vi "parse load from file.vi"(8 "error in":errorcluster, 11 "message data":string) -> (0 "error out":errorcluster, 2 "targets to load":string[](array[string]), 3 "path":path)   [LabVIEW 2013, in "module execution process.lvlib"]
uses:
  module execution process.lvlib
  tokenized path.ctl
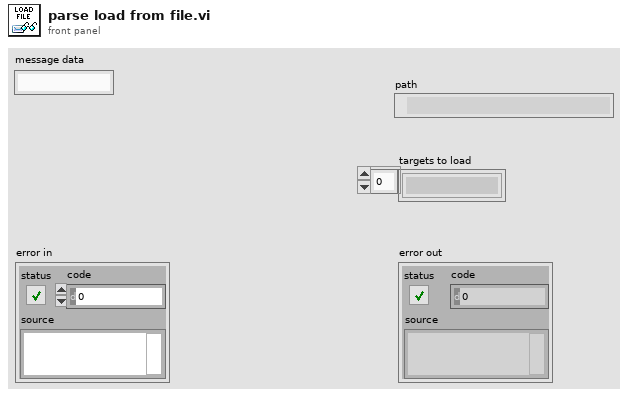
[diagram p1: front panel]
types:
  T1 = typedef "module execution process.lvlib/tokenized path.ctl" = string[]
  T2 = cluster{"tokenized path":T1, "targets to load":string[]}
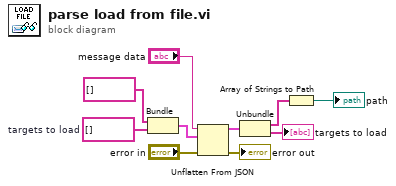
[diagram p0: block diagram]
diagram:
  w7 = string[] []  # targets to load
  n1 = Bundle("tokenized path"=T1 [], "targets to load"=w7) -> (w6:T2)  [unwired: 1 in]
  n2 = Unflatten From JSON(JSON string="message data", type and defaults=w6, error in (no error)="error in") -> (value=w5:T2, error out=→"error out":errorcluster)  [unwired: 4 in]
  n3 = Unbundle(w5) -> ("tokenized path"=w3:T1, "targets to load"=→"targets to load":string[])
  n4 = Array of Strings to Path(0:w3) -> (2:→"path":path)  [unwired: 1 in]
